vi "write_attributes.vi"(8 "error in (no error)":errorcluster, 10 "attributes":T1, 11 "QuadraticDiscriminantAnalysis in":refnum<class "QuadraticDiscriminantAnalysis.lvclass">) -> (0 "error out":errorcluster, 3 "QuadraticDiscriminantAnalysis out":refnum<class "QuadraticDiscriminantAnalysis.lvclass">)   [LabVIEW 2020, in "QuadraticDiscriminantAnalysis.lvclass"]
uses:
  QuadraticDiscriminantAnalysis.lvclass
  Controls/quadratic_discriminant_analysis_attributes.ctl
  QuadraticDiscriminantAnalysis.lvclass/QuadraticDiscriminantAnalysis.ctl
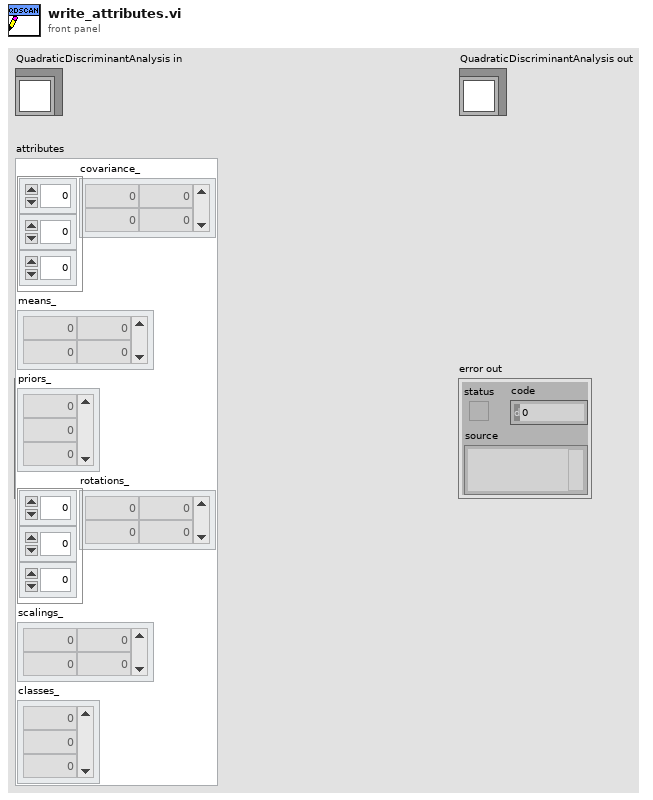
[diagram p1: front panel]
types:
  T1 = typedef "quadratic_discriminant_analysis_attributes.ctl" = cluster{"covariance_":dbl[][][], "means_":dbl[][], "priors_":dbl[], "rotations_":dbl[][][], "scalings_":dbl[][], "classes_":dbl[]}
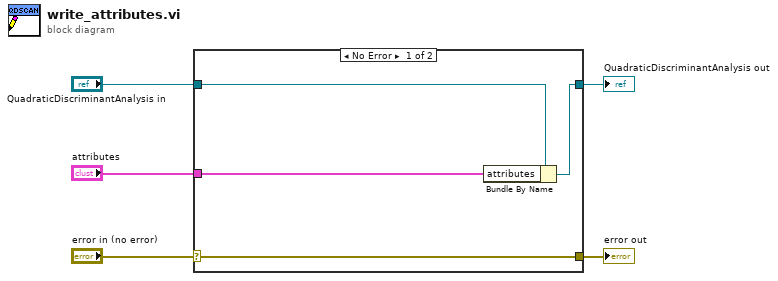
[diagram p0: block diagram]
diagram:
  n1 = case shown="No Error" "error in (no error)" {
    selector: "error in (no error)" -> [w9 w10]
    tunnel: [w9 w10] -> w4
    tunnel: [w7 w11] -> w2
    tunnel: "QuadraticDiscriminantAnalysis in" -> [w8 w11]
    tunnel: "attributes" -> [w6 _]
    frame No Error {
      n2 = Bundle By Name(cluster=w8, "attributes"=w6) -> (w7:refnum<class "QuadraticDiscriminantAnalysis.lvclass">)
    }
    frame Error {
    }
  }
  "error out" <- w4
  "QuadraticDiscriminantAnalysis out" <- w2
